vi "Add Messages and Subaddresses from Definitions.vi"(8 "error in":errorcluster, 10 "message definitions":T1[](array[typedef]), 11 "port":T6 format="%.0x") -> (0 "error out":errorcluster, 3 "port out":T6 format="%.0x")   [LabVIEW 2020, in "AIM MIL-STD-1553 Scripting.lvlib"]
doc: "Adds Messages and associated Subaddresses to Terminals within the <b>port</b> as defined in <b>message configurations</b>."
uses:
  AIM MIL-STD-1553 Scripting.lvlib
  <vilib>/NI VeriStand/Custom Device API/Custom Device Item Ref.ctl
  Shared/Message Definition.ctl
  Shared/Message Type.ctl
  Shared/Terminal Endpoint.ctl
  Shared/Address.ctl
  Shared/Parameter Definition.ctl
  <vilib>/NI VeriStand/Custom Device API/Custom Device API.lvlib
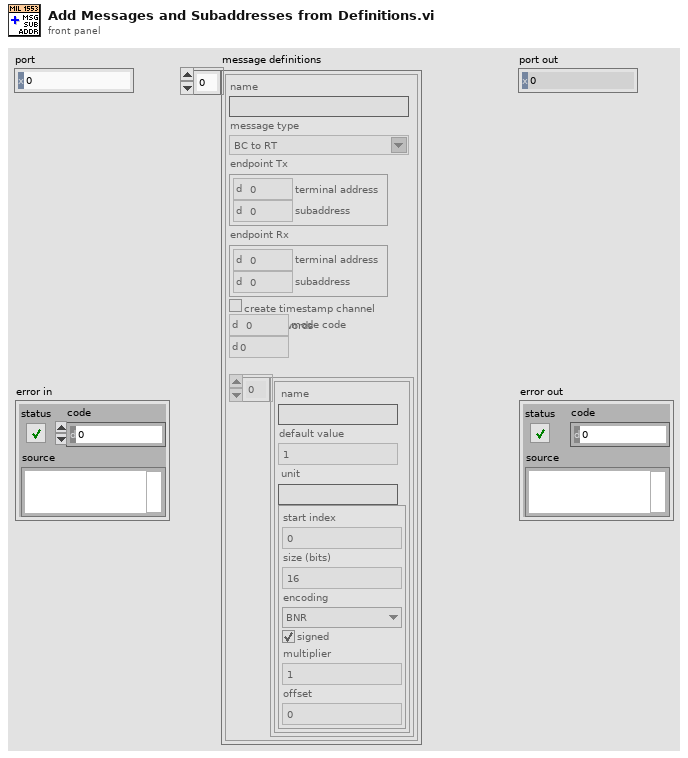
[diagram p1: front panel]
types:
  T1 = typedef "Message Definition.ctl" = cluster{"name":string, "message type":T2, "endpoint Tx":T3, "endpoint Rx":T3, "create timestamp channel":bool, "mode code":u16, "number of words":u16, "parameters":cluster{"name":string, "default value":dbl, "unit":string, "parameter definition":T5}[]}
  T2 = typedef "Message Type.ctl" = string
  T3 = typedef "Terminal Endpoint.ctl" = cluster{"terminal address":T4, "subaddress":T4}
  T4 = typedef "Address.ctl" = u16
  T5 = typedef "Parameter Definition.ctl" = cluster{"start index":i32, "size (bits)":i32, "encoding":enum16{"BNR", "BCD", "Discrete"}, "signed":bool, "multiplier":dbl, "offset":dbl}
  T6 = typedef "Custom Device API.lvlib/Custom Device Item Ref.ctl" = u64
  T7 = cluster{"name":string, "default value":dbl, "unit":string, "parameter definition":T5}[]
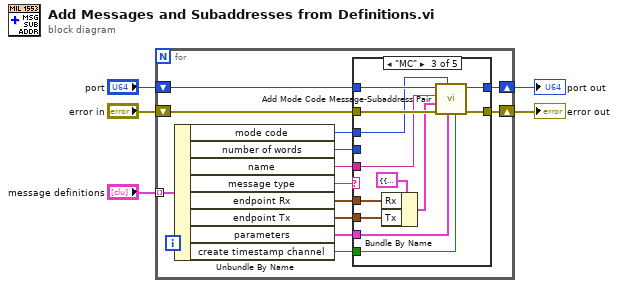
[diagram p0: block diagram]
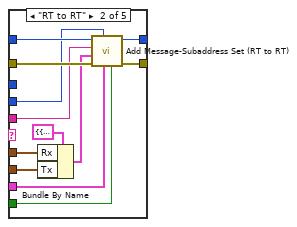
[diagram p3: hidden frame]
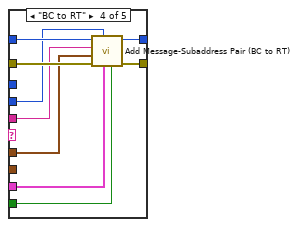
[diagram p4: hidden frame]
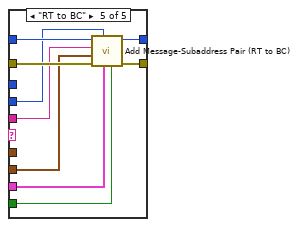
[diagram p5: hidden frame]
diagram:
  n1 = for {
    tunnel: "message definitions" -> [w9] mode=indexing
    shift-right: [w10] -> w2
    shift-left: "error in" -> [w11]
    shift-right: [w7] -> w3
    shift-left: "port" -> [w12]
    n2 = Unbundle By Name(w9) -> ("mode code"=w6:u16, "number of words"=w8:u16, "name"=w17:string, "message type"=w18:T2, "endpoint Rx"=w16:T3, "endpoint Tx"=w15:T3, "parameters"=w14:T7, "create timestamp channel"=w13:bool)
    n3 = case shown="\"MC\"" w18 {
      tunnel: w17 -> [_ w29 w42 w49 w58]
      tunnel: w16 -> [_ w27 w40 w48 _]
      tunnel: w15 -> [_ w26 w39 _ w54]
      tunnel: w14 -> [_ w24 w37 w47 w57]
      tunnel: w13 -> [_ w23 w36 w46 w56]
      tunnel: w12 -> [w19 w32 w44 w53 w62]
      tunnel: w11 -> [w20 w31 w43 w52 w61]
      tunnel: [w20 w22 w35 w51 w60] -> w10
      tunnel: w8 -> [_ w30 _ w50 w59]
      tunnel: [w19 w21 w34 w45 w55] -> w7
      tunnel: w6 -> [_ _ w33 _ _]
      frame Default {
      }
      frame "RT to RT" {
        n4 = Bundle By Name(cluster=cluster{"Rx":T3, "Tx":T3} {"Rx"={"terminal address"=0, "subaddress"=0}, "Tx"={"terminal address"=0, "subaddress"=0}} ("remote terminals"), "Rx"=w27, "Tx"=w26) -> (w25:cluster{"Rx":T3, "Tx":T3})
        n5 = call "Add Message-Subaddress Set (RT to RT).vi"("create timestamp channel"=w23, "parameters"=w24, "number of words"=w30, "error in"=w31, "remote terminals"=w25, "name"=w29, "port"=w32) -> ("error out"=w22:errorcluster, "port out"=w21:T6)  [unwired: 2 in, 1 out]
      }
      frame "MC" {
        n6 = Bundle By Name(cluster=cluster{"Rx":T3, "Tx":T3} {"Rx"={"terminal address"=0, "subaddress"=0}, "Tx"={"terminal address"=0, "subaddress"=0}} ("remote terminals"), "Rx"=w40, "Tx"=w39) -> (w38:cluster{"Rx":T3, "Tx":T3})
        n7 = call "Add Mode Code Message-Subaddress Pair.vi"("create timestamp channel"=w36, "parameters"=w37, "mode code"=w33, "error in"=w43, "terminals"=w38, "name"=w42, "port"=w44) -> ("error out"=w35:errorcluster, "port out"=w34:T6)  [unwired: 1 in, 2 out]
      }
      frame "BC to RT" {
        n8 = call "Add Message-Subaddress Pair (BC to RT).vi"("create timestamp channel"=w46, "parameters"=w47, "number of words"=w50, "error in"=w52, "rx remote terminal"=w48, "name"=w49, "port"=w53) -> ("error out"=w51:errorcluster, "port out"=w45:T6)  [unwired: 1 in, 2 out]
      }
      frame "RT to BC" {
        n9 = call "Add Message-Subaddress Pair (RT to BC).vi"("create timestamp channel"=w56, "parameters"=w57, "number of words"=w59, "error in"=w61, "tx remote terminal"=w54, "name"=w58, "port"=w62) -> ("error out"=w60:errorcluster, "port out"=w55:T6)  [unwired: 1 in, 2 out]
      }
    }
  }
  "error out" <- w2
  "port out" <- w3
